vi "DrawBigDigit.vi"(6 "color":fxp<+,3,3>, 8 "error in (no error)":errorcluster, 9 "Digit":i32, 10 "Position":T1) -> (0 "error out":errorcluster)   [LabVIEW 2019, in "RT_Game.lvlib" / "Engine.lvclass"]
uses:
  Engine.lvclass
  Coordinate.ctl
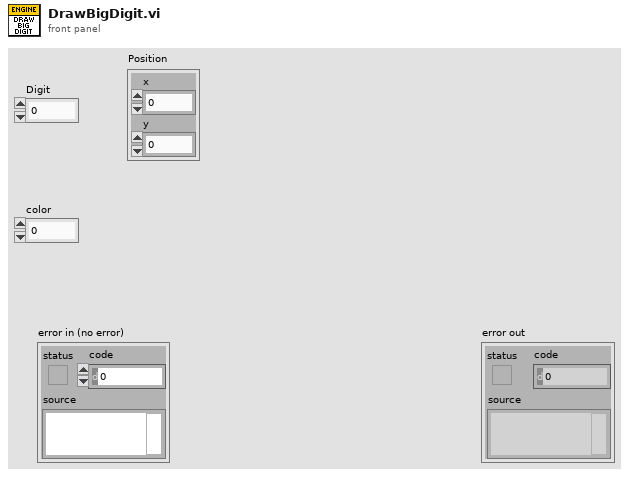
[diagram p1: front panel]
types:
  T1 = typedef "RT_Game.lvlib/Engine.lvclass/Coordinate.ctl" = cluster{"x":dbl, "y":dbl}
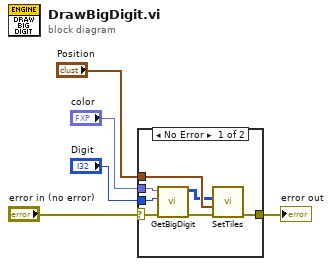
[diagram p0: block diagram]
diagram:
  n1 = case shown="No Error" "error in (no error)" {
    selector: "error in (no error)" -> [w12 w13]
    tunnel: [w11 w13] -> w4
    tunnel: "Digit" -> [w10 _]
    tunnel: "Position" -> [w9 _]
    tunnel: "color" -> [w8 _]
    frame No Error {
      n2 = call "GetBigDigit.vi"("error in (no error)"=w12, "Digit"=w10, "color"=w8) -> ("error out"=w7:errorcluster, "Array"=w6:u32[][])  [unwired: 7 in]
      n3 = call "SetTiles.vi"("error in (no error)"=w7, "Position"=w9, "TileCodes"=w6) -> ("error out"=w11:errorcluster)  [unwired: 8 in]
    }
    frame Error {
    }
  }
  "error out" <- w4
